vi "InitFromConfiguration.vi"(4 "configuration":T1) -> (1 "output cluster":T1)   [LabVIEW 2017]
uses:
  <vilib>/Utility/tdmsutil.llb/fileViewerConfigData.ctl
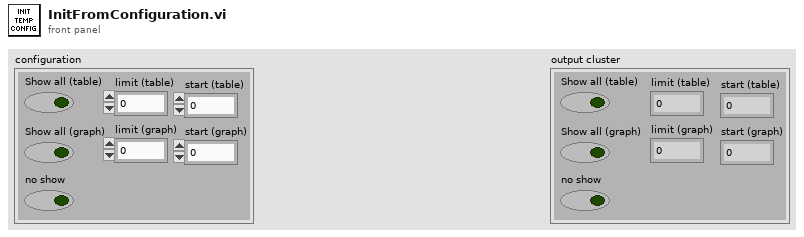
[diagram p1: front panel]
types:
  T1 = typedef "fileViewerConfigData.ctl" = cluster{"Show all (table)":bool, "Show all (graph)":bool, "limit (table)":u64, "limit (graph)":u64, "no show":bool, "start (table)":u64, "start (graph)":u64}
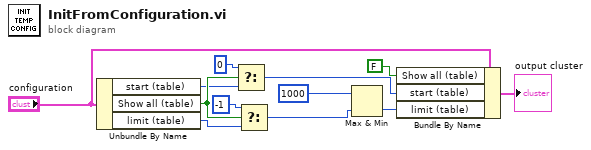
[diagram p0: block diagram]
diagram:
  n1 = Unbundle By Name("configuration") -> ("start (table)"=w10:u64, "Show all (table)"=w11:bool, "limit (table)"=w12:u64)
  n2 = Select(t=u64 0, s=w11, f=w10) -> (s? t:f=w4:u64)
  n3 = Select(t=i64 -1 ("count (-1: all)"), s=w11, f=w12) -> (s? t:f=w6:u64)
  n4 = Max & Min(x=u64 1000 ("y"), y=w6) -> (min(x,y)=w3:u64)  [unwired: 1 out]
  n5 = Bundle By Name(cluster="configuration", "Show all (table)"=FALSE, "start (table)"=w4, "limit (table)"=w3) -> (→"output cluster":T1)
